vi "1. VI PRINCIPAL XXX XXX V1.vi"() -> ()   [LabVIEW 2019]
panel:
  in  "Stop Button":bool
  in  "Menú":enum32{"Edición", "Reporte"}(tab)
  in  "Tab Control":T1(tab)
  out "Horizontal Pointer Slide 2":dbl
  in  "+":bool
  in  "-":bool
  out "+ 2":bool
  out "- 2":bool
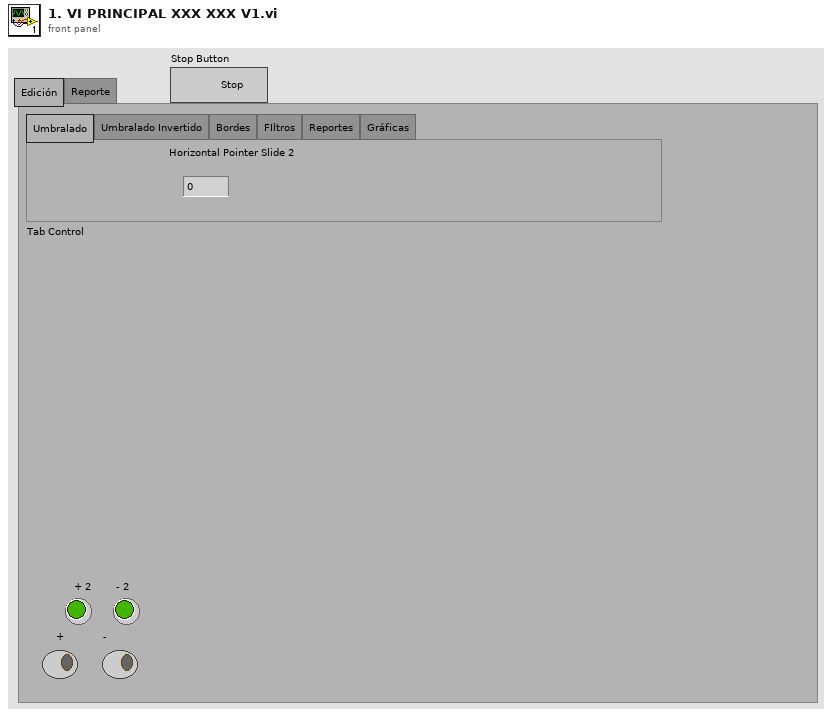
[diagram p1: front panel]
types:
  T1 = enum32{"Umbralado", "Umbralado Invertido", "Bordes", "FIltros", "Reportes", "Gráficas"}
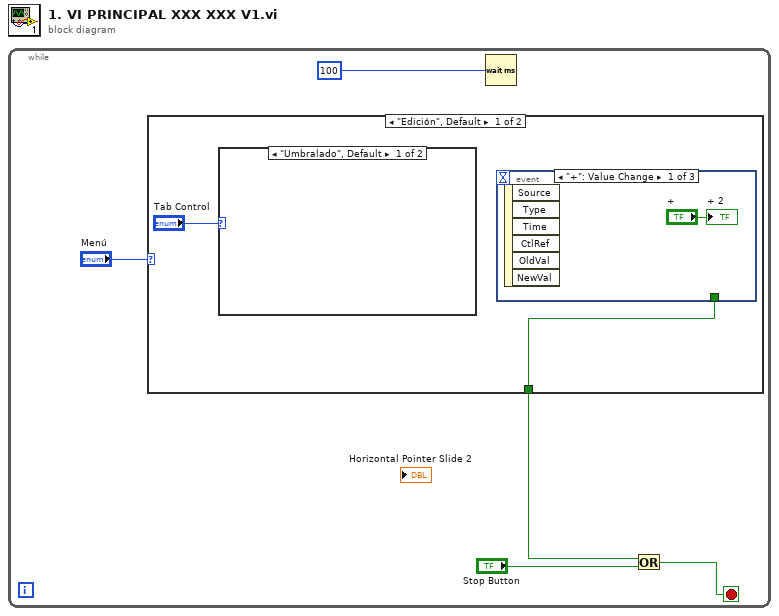
[diagram p0: block diagram]
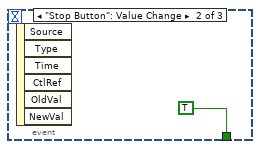
[diagram p2: hidden frame]
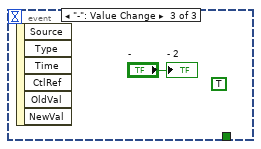
[diagram p3: hidden frame]
diagram:
  n1 = while {
    stop <- w3 stop-if-true
    n2 = case shown="\"Edición\", Default" "Menú" {
      tunnel: [w6 _] -> w1
      frame "Edición", Default {
        n3 = case shown="\"Umbralado\", Default" "Tab Control" {
          frame "Umbralado", Default {
          }
          frame "Bordes" {
          }
        }
        n4 = event shown="[0] \"+\": Value Change" {
          selector: _ -> [_ _ _]
          dyn-events: _ -> [_ _ _]
          timeout: _ -> [_ _ _]
          tunnel: [_ TRUE _] -> w6
          event "+": Value Change {
            n5 = event-data() -> ()  [unwired: 1 in, 6 out]
            "+ 2" <- "+"
          }
          event "Stop Button": Value Change {
            n6 = event-data() -> ()  [unwired: 1 in, 6 out]
          }
          event "-": Value Change {
            (unwired) TRUE
            n7 = event-data() -> ()  [unwired: 1 in, 6 out]
            "- 2" <- "-"
          }
        }
      }
      frame "Reporte" {
      }
    }
    n8 = Wait (ms)(milliseconds to wait=u32 100) -> ()  [unwired: 1 out]
    n9 = Or(x=w1, y="Stop Button") -> (x .or. y?=w3:bool)
  }
